vi "VNA and Opticool.vi"() -> ()   [LabVIEW 2024]
uses:
  <vilib>/Analysis/baseanly.llb/Mean (DBL).vi
  <vilib>/Utility/file.llb/Write Delimited Spreadsheet (DBL).vi
  <vilib>/Analysis/NI_AALBase.lvlib
  D:/LabData/Fan Fei/VNA/Agilent ENA Series/Agilent ENA Series.lvlib
panel:
  in  "file path":path=path "C:/Users/Public/OneDrive/Desktop/test/textR.txt"
  out "variance":dbl format="%0.2f"
  out "standard deviation":dbl format="%0.2f"
  out "mean":dbl=9.900000302096328e+37 format="%0.2f"
  in  "Num Meas":u32=10
  in  "Compliance  Level (0.1)":dbl=0.001
  in  "Source Mode  (0: Voltage)":u16(ring) items=["Voltage", "Current"]
  in  "Output Level (0)":dbl=3.0
  in  "VISA resource name 2":refnum<visa-resource-name>="GPIB0::18::INSTR"
  in  "stop":bool
  in  "file path (dialog if empty) Scan 2":path=path "C:/Users/B1172_SHG/Documents/NOEMS/test.txt"
  in  "Second Scan":bool
  in  "Port ( 1)  2":i32=1
  in  "Measurement Parameters   2":u16(ring)=1 items=["S11", "S21", "S31", "S41", "S12", "S22", "S32", "S42", "S13", "S23", "S33", "S43", "S14", "S24", "S34", "S44", "A", "B", "C", "D", "R1", "R2", "R3", "R4"]
  in  "Power Level (dBm)  2":dbl=-5.0 format="%^.2g"
  in  "VNA Points  2":i32=1000
  in  "Start (Mhz)  2":dbl=1.0 format="%^.2e"
  in  "Stop (MHz)  2":dbl=10.0 format="%^.2e"
  in  "Trigger Source   2":u16(ring) items=["Internal", "External", "Manual", "BUS"]
  in  "Point Trigger (F: Disable) 3":bool
  in  "Continuous Sweep (T: Enable)  2":bool=TRUE
  in  "Averaging State (F: Off) 3":bool
  in  "Average Factor (16) 3":i32=16
  in  "IF Bandwidth (100000.0)  2":dbl=1000.0 format="%^.1e"
  in  "Smoothing State (F: Off) 3":bool
  in  "Wait time (ms)  2":dbl=4000.0
  out "XY Graph 3":cluster{dbl[], "Primary / Real":dbl[]}(graph)
  in  "Continue":bool
  in  "Field Set when finsihed":dbl
  in  "Port ( 1)":i32=1
  in  "Measurement Parameters":u16(ring)=1 items=["S11", "S21", "S31", "S41", "S12", "S22", "S32", "S42", "S13", "S23", "S33", "S43", "S14", "S24", "S34", "S44", "A", "B", "C", "D", "R1", "R2", "R3", "R4"]
  in  "Power Level (dBm)":dbl=-5.0 format="%^.2g"
  in  "VNA Points":i32=1000
  in  "Start (Mhz)":dbl=1.0 format="%^.2e"
  in  "Stop (MHz)":dbl=10.0 format="%^.2e"
  in  "Trigger Source":u16(ring) items=["Internal", "External", "Manual", "BUS"]
  in  "Point Trigger (F: Disable) 2":bool
  in  "Continuous Sweep (T: Enable)":bool=TRUE
  in  "Averaging State (F: Off) 2":bool
  in  "Average Factor (16) 2":i32=16
  in  "IF Bandwidth (100000.0)":dbl=1000.0 format="%^.1e"
  in  "Smoothing State (F: Off) 2":bool
  in  "Wait time (ms)":dbl=4000.0
  out "XY Graph 2":cluster{dbl[], "Primary / Real":dbl[]}(graph)
  in  "T scan waiting time (min)":dbl
  in  "Scan T":bool=TRUE
  in  "T Step Size":dbl=10.0
  in  "Start B":dbl
  in  "B Step Size":dbl
  in  "B Number of Step":i32=1
  in  "Start T":dbl=300.0
  in  "T Number of Step":i32=20
  in  "Temperature Set when finish":dbl=300.0
  in  "file path (dialog if empty)":path=path "C:/Users/Public/OneDrive/Desktop/test/text.txt"
  in  "VISA resource name":refnum<visa-resource-name>="GPIB0::27::INSTR"
  in  "Remote":bool=TRUE
  in  "IP Address":string="169.254.170.239"
  out "Measuring":bool=TRUE
  out "Temperature":dbl=300.0
  in  "WaitForTemperature":bool=TRUE
  in  "WaitForField":bool=TRUE
  in  "Delay":dbl=5.0
  out "Field":dbl
  out "Field\nStatus":i32(ring)=4 items=["MagnetUnknown"=0, "StablePersistent"=1, "WarmingSwitch"=2, "CoolingSwitch"=3, "StableDriven"=4, "Iterating"=5, "Charging"=6, "Discharging"=7, "CurrentError"=8, "MagnetFailure"=15]
  out "Temperature\nStatus":i32(ring)=1 items=["TemperatureUnknown"=0, "Stable"=1, "Tracking"=2, "Near"=5, "Chasing"=6, "Filling"=7, "Standby"=10, "Disabled"=13, "ImpedanceNotFunction"=14, "TempFailure"=15]
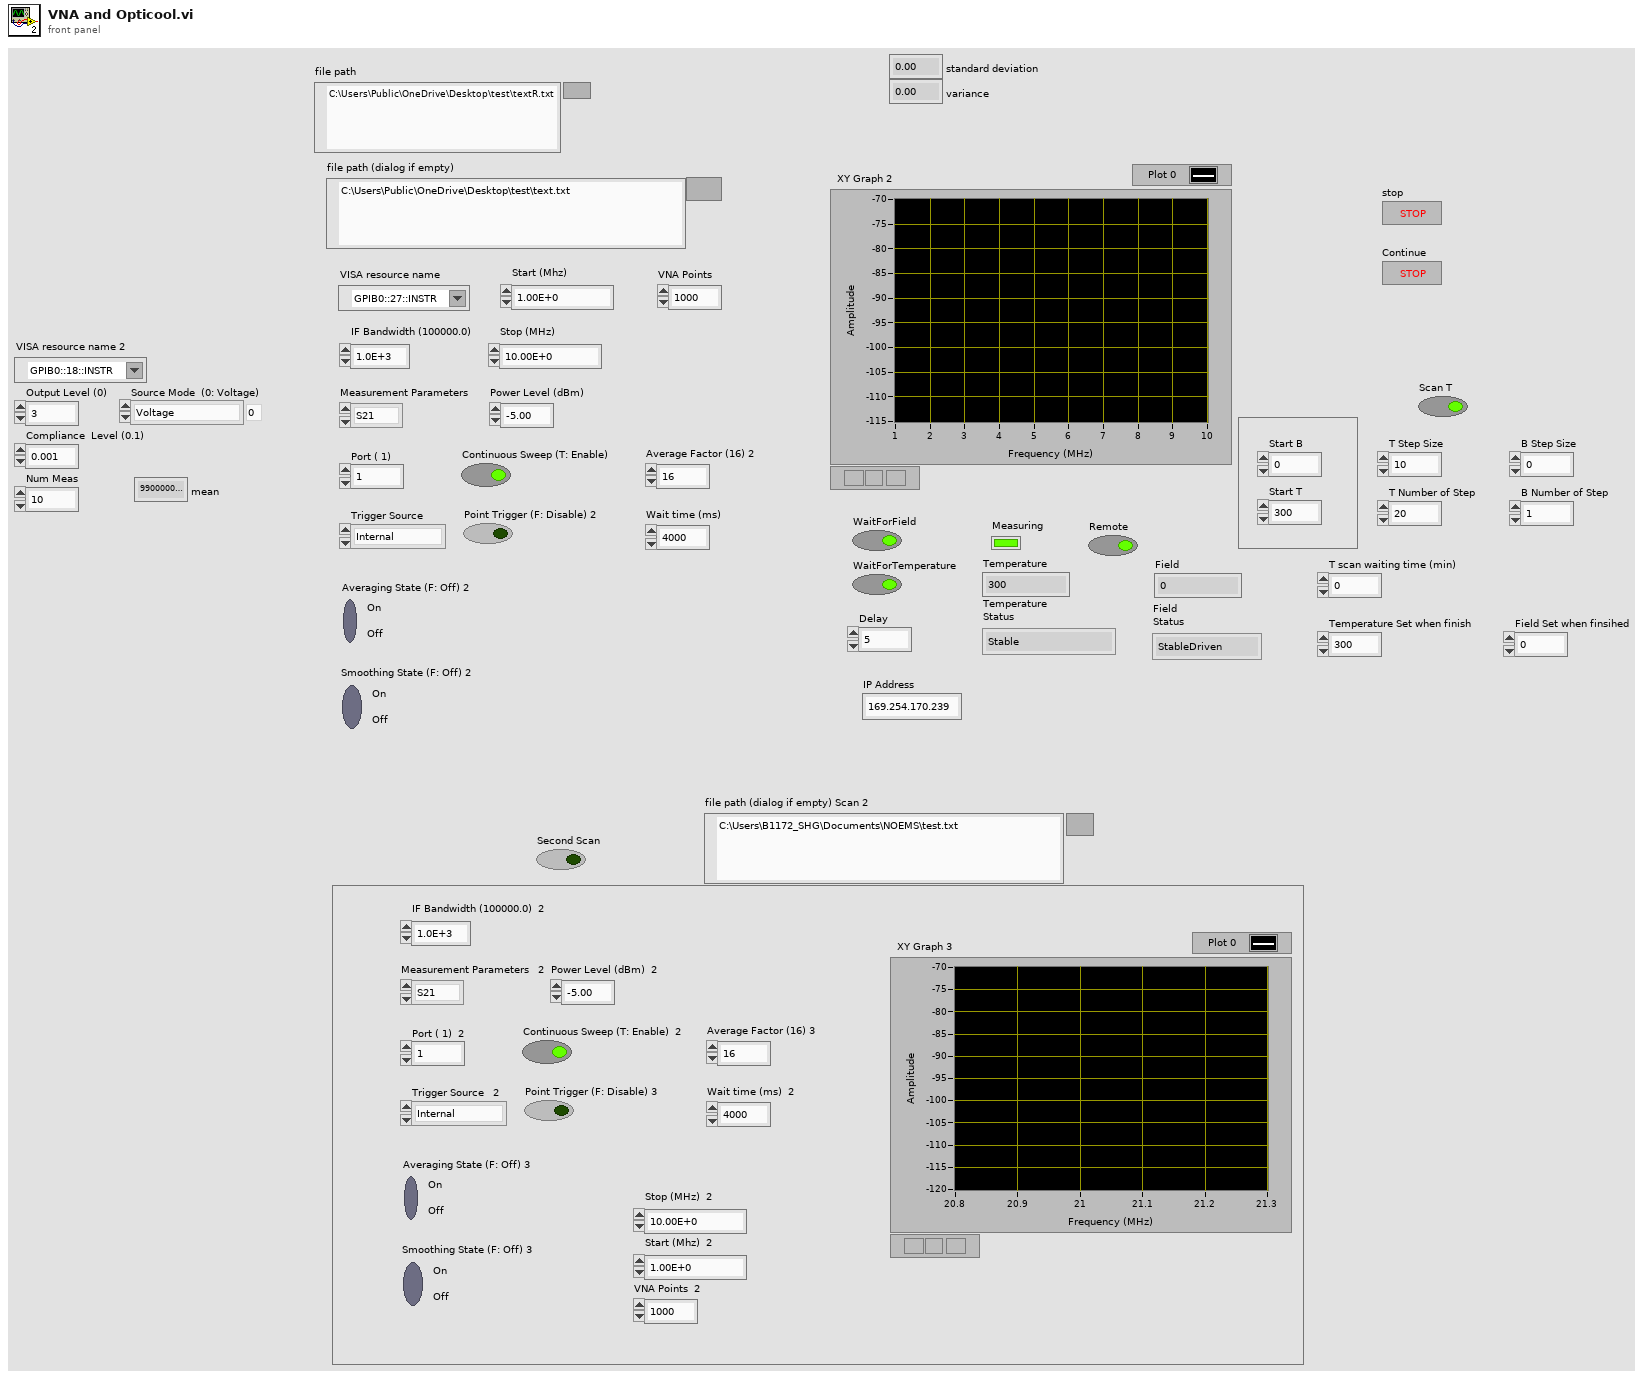
[diagram p1: front panel]
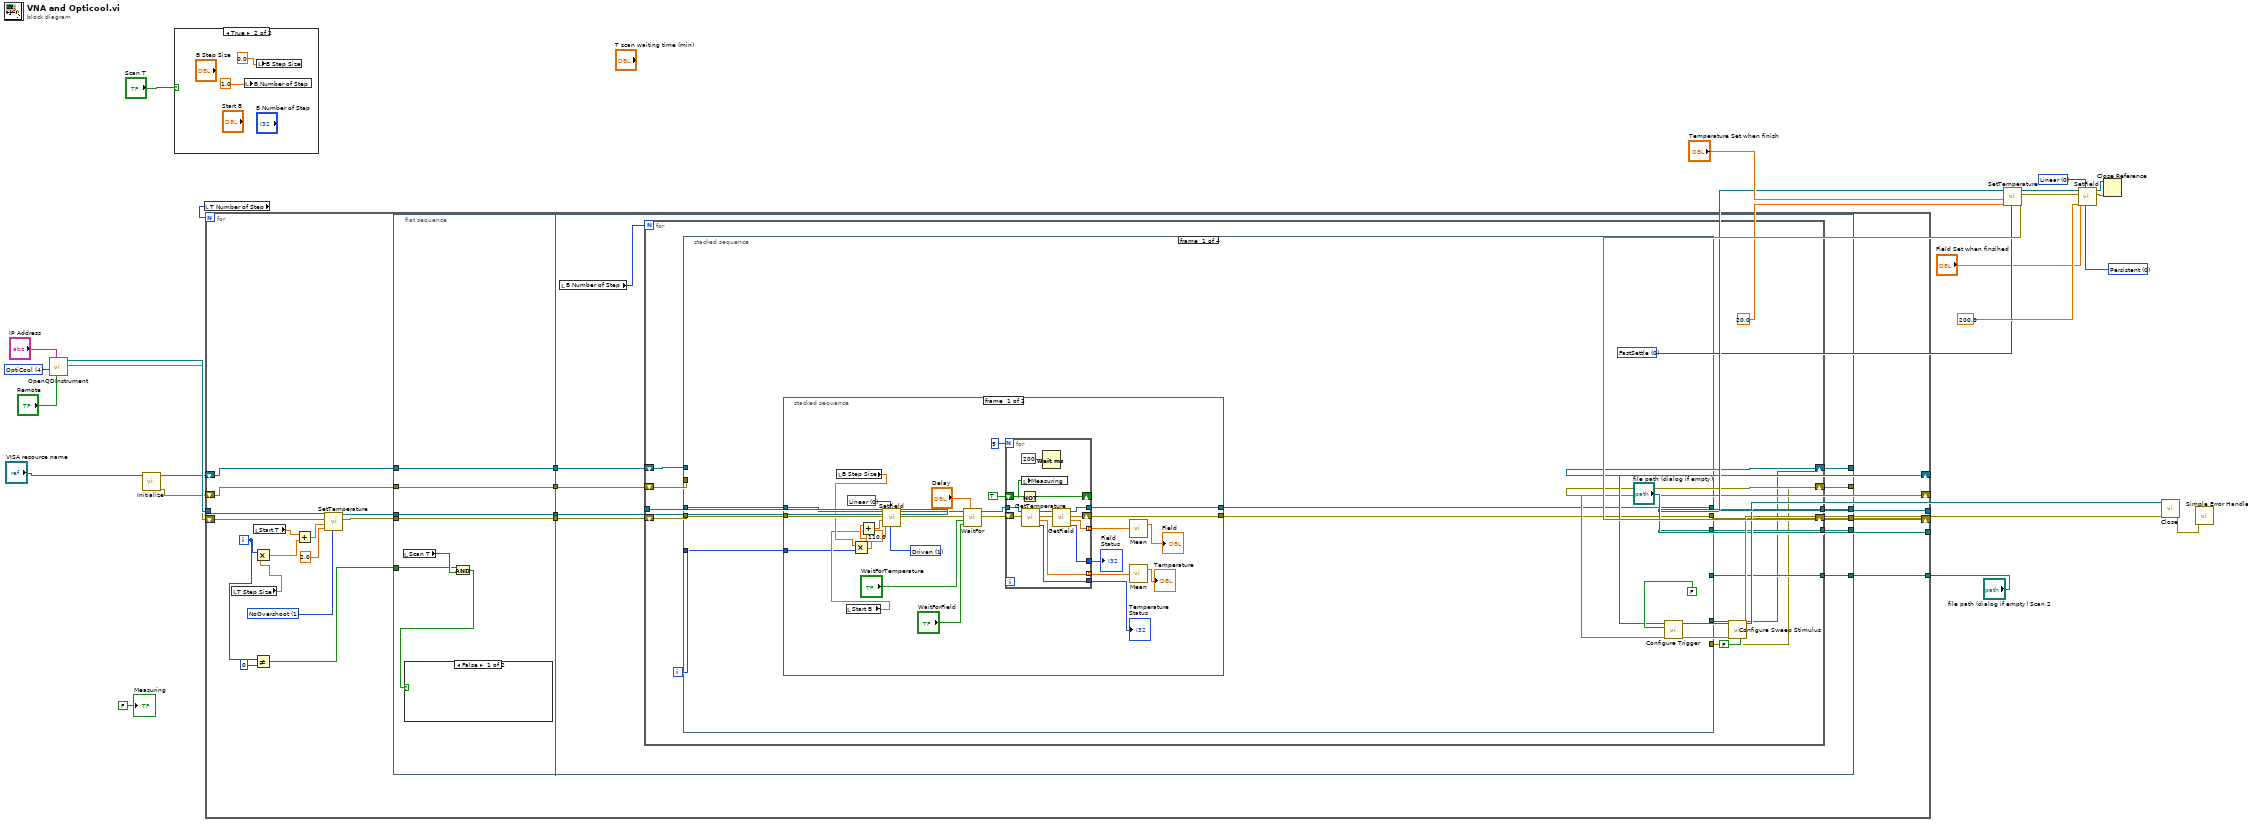
[diagram p0: block diagram]
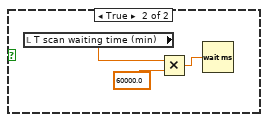
[diagram p2: hidden frame]
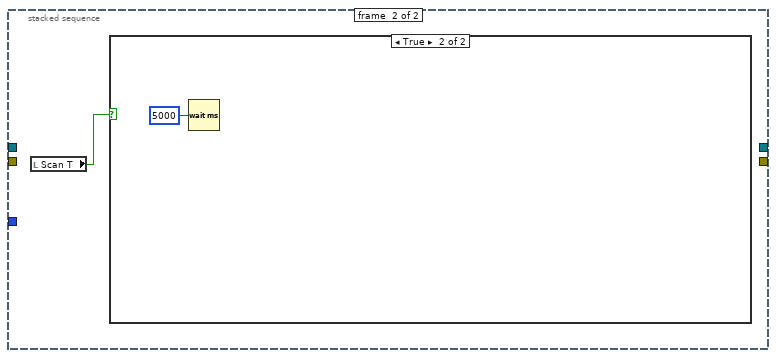
[diagram p3: hidden frame]
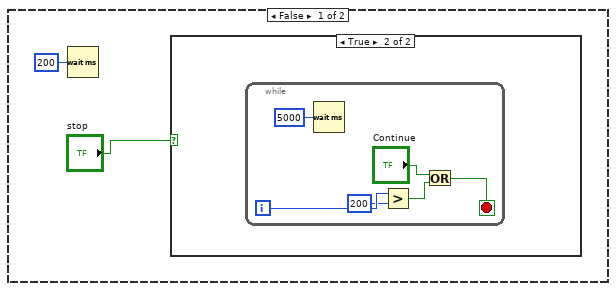
[diagram p4: hidden frame]
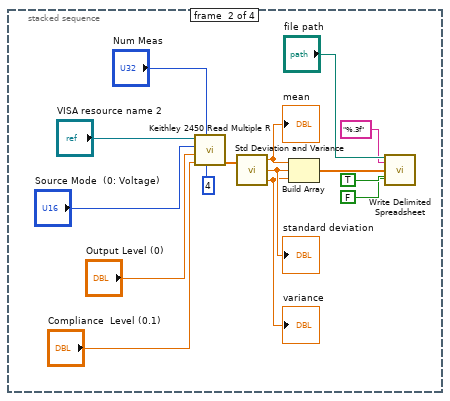
[diagram p6: hidden frame]
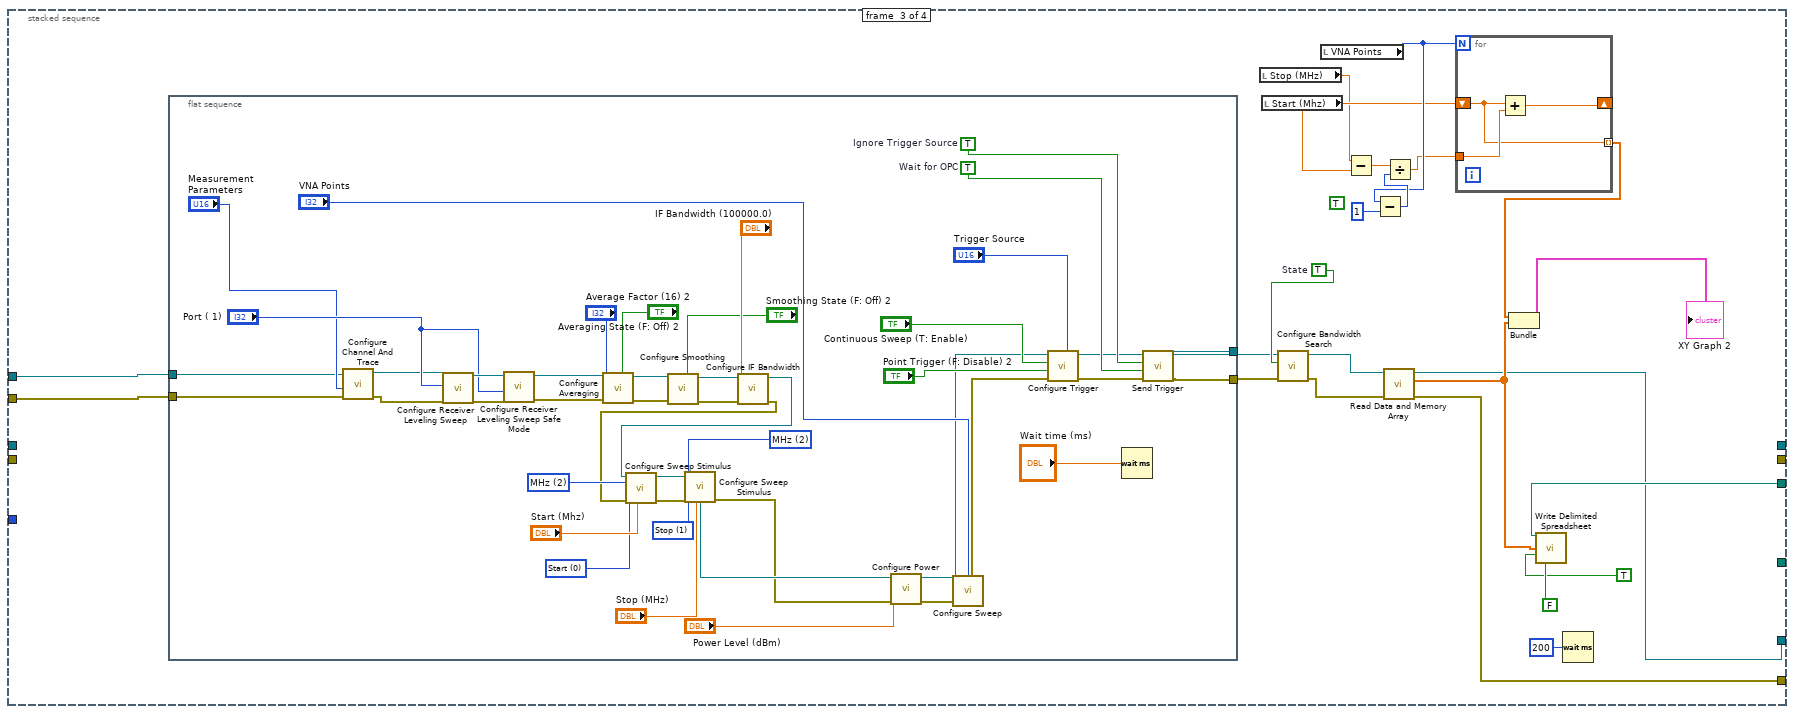
[diagram p7: hidden frame]
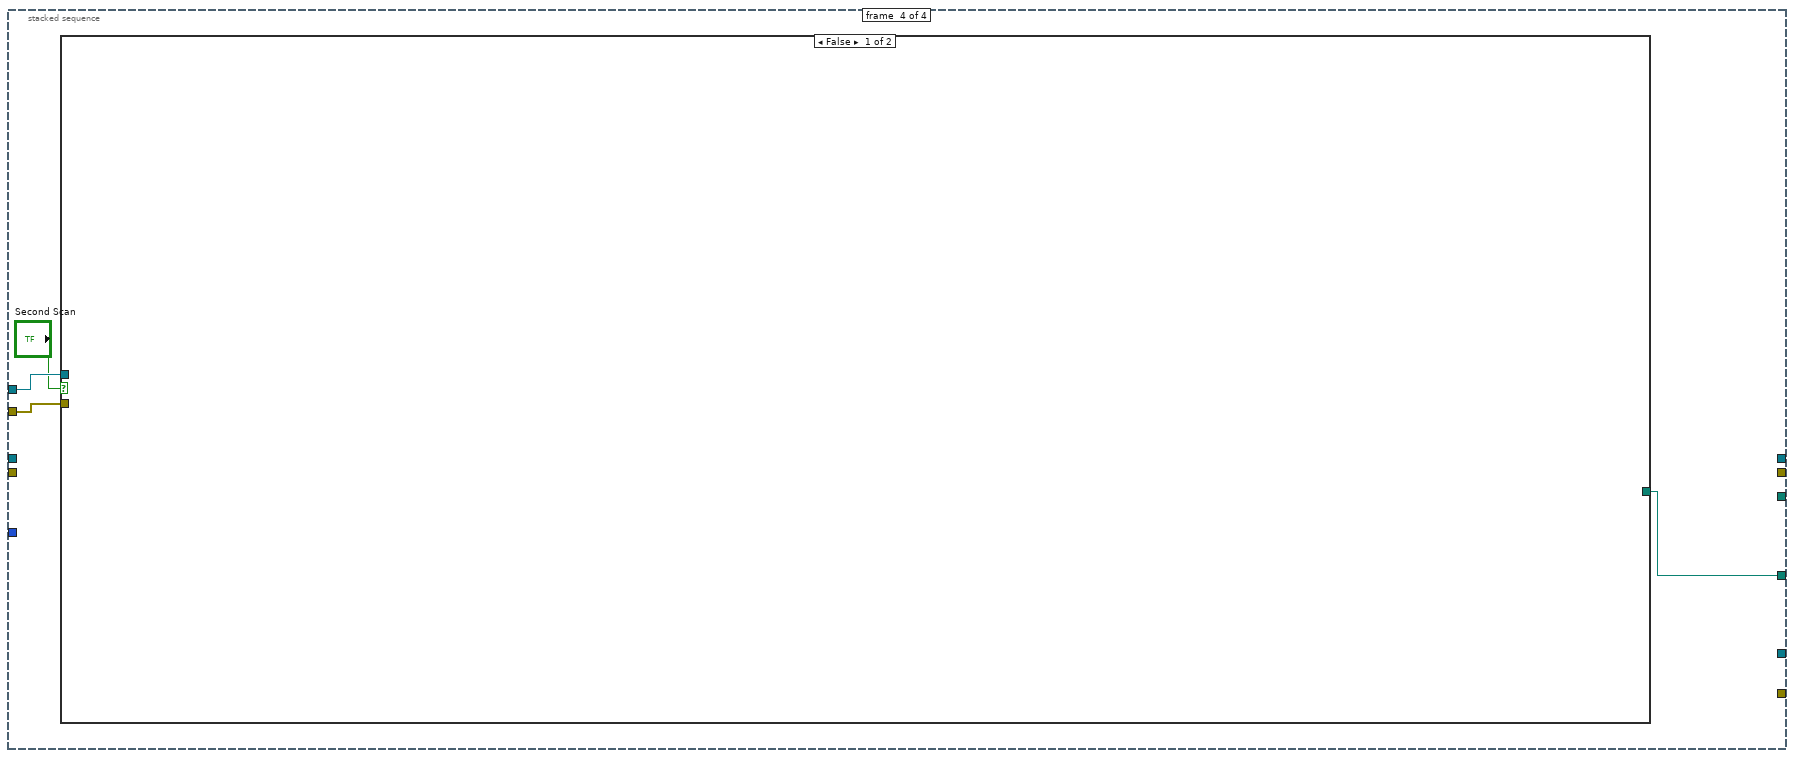
[diagram p8: hidden frame]
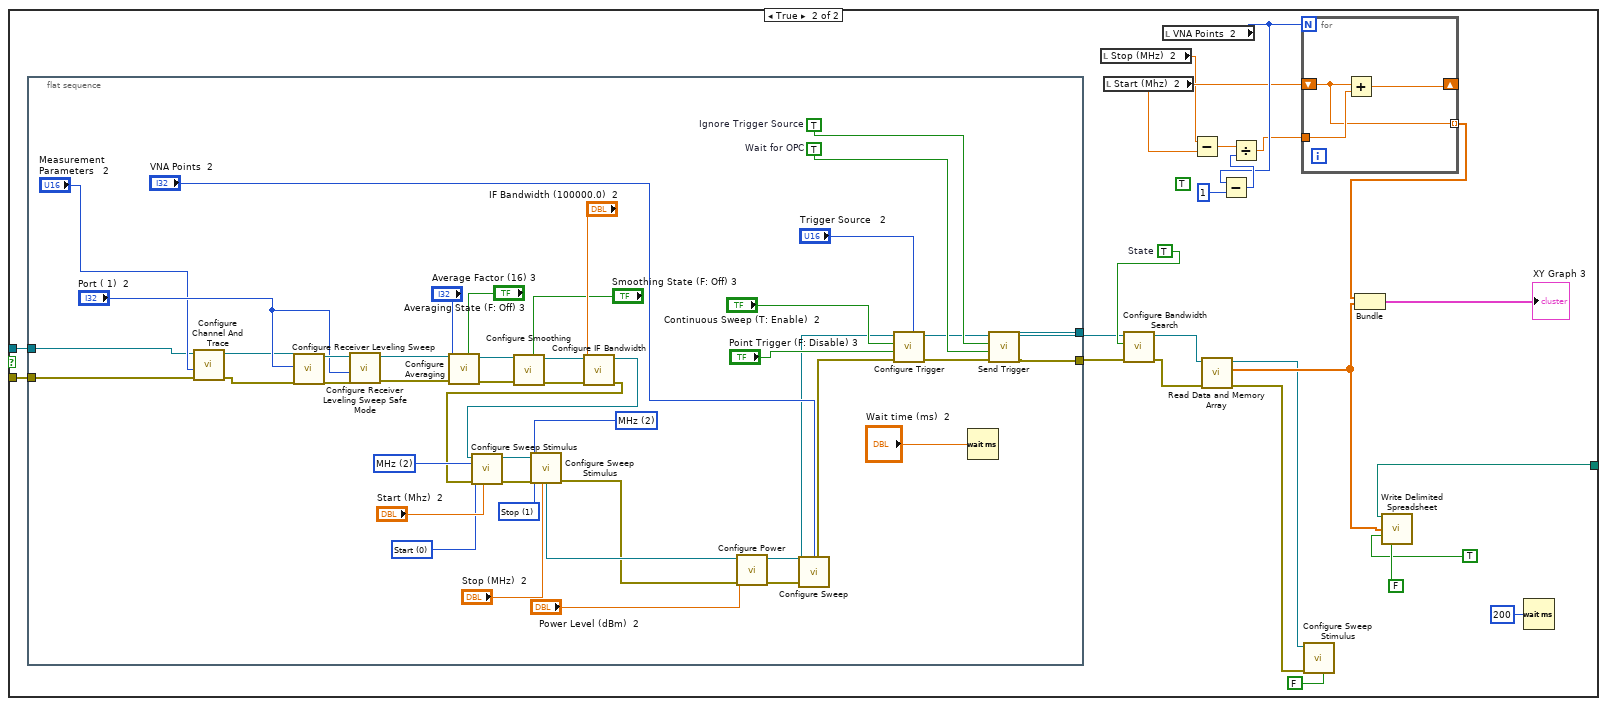
[diagram p9: hidden frame]
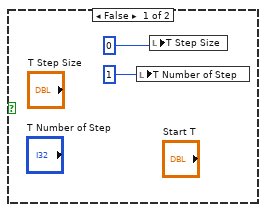
[diagram p10: hidden frame]
diagram:
  w18 = 0 items=["FastSettle", "NoOvershoot"] ("Approach")
  w21 = 4 items=["PPMS", "VersaLab", "DynaCool", "SVSM", "OptiCool"] ("InstrumentType")
  w33 = 0 items=["Persistent", "Driven"] ("Mode")
  w32 = 0 items=["Linear", "NoOvershoot", "Oscillate"] ("Approach")
  n1 = call "OpenQDInstrument.vi"("Remote"="Remote", "IP Address"="IP Address", "InstrumentType"=w21) -> ("error out"=w19:errorcluster, "Instrument Ref"=w20:refnum<k24>)  [unwired: 5 in]
  n2 = call "Initialize.vi"("VISA resource name"="VISA resource name") -> ("error out"=w3:errorcluster, "VISA resource name out"=w5:refnum<visa-resource-name>)  [unwired: 9 in]
  n3 = case shown="True" "Scan T" {
    frame False {
      n4 = local write "T Number of Step"(1) -> ()
      n5 = local write "T Step Size"(0) -> ()
    }
    frame True {
      n6 = local write "B Number of Step"(1.0 ("B Step Size")) -> ()
      n7 = local write "B Step Size"(0.0 ("B Step Size")) -> ()
    }
  }
  n8 = local read "T Number of Step"() -> (w8:i32)
  n9 = for {
    N: w8 -> [_]
    shift-right: [w58] -> w27
    shift-left: w19 -> [w62]
    tunnel: w20 -> [w61]
    tunnel: [w56] -> w24
    tunnel: "file path (dialog if empty)" -> [w52]
    shift-right: [w51] -> w7
    shift-left: w5 -> [w49]
    shift-right: [w50] -> w4
    shift-left: w3 -> [w48]
    tunnel: "file path (dialog if empty) Scan 2" -> [w43]
    i -> [w42]
    w57 = 1 items=["FastSettle", "NoOvershoot"] ("Approach")
    n10 = local read "T Step Size"() -> (w53:dbl)
    n11 = local read "Start T"() -> (w54:dbl)
    n12 = Multiply(x=w42, y=w53) -> (x*y=w55:dbl)
    n13 = Not Equal?(x=w42, y=0) -> (x != y?=w40:bool)
    n14 = Add(x=w54, y=w55) -> (x+y=w64:dbl)
    n15 = call "SetTemperature.vi"("Approach"=w57, "Rate"=2.0, "Temperature"=w64, "error in (no error)"=w62, "Instrument Ref In"=w61) -> ("error out"=w59:errorcluster, "Instrument Ref Out"=w60:refnum<k24>)  [unwired: 2 in, 1 out]
    n16 = flat-sequence {
      tunnel: w48 -> [w68]
      tunnel: w49 -> [w69]
      tunnel: w59 -> [w70]
      tunnel: w60 -> [w71]
      tunnel: [w71] -> w47
      tunnel: [w70] -> w46
      tunnel: [w69] -> w45
      tunnel: [w68] -> w44
      tunnel: w40 -> [w66]
      tunnel: [w83] -> w58
      tunnel: [w82] -> w56
      tunnel: w52 -> [w80]
      tunnel: [w79] -> w51
      tunnel: [w78] -> w50
      tunnel: w47 -> [w85]
      tunnel: w46 -> [w84]
      tunnel: w45 -> [w77]
      tunnel: w44 -> [w76]
      tunnel: w43 -> [w75]
      frame #0 {
        n17 = local read "Scan T"() -> (w67:bool)
        n18 = And(x=w66, y=w67) -> (x .and. y?=w65:bool)
        n19 = case shown="False" w65 {
          frame False {
          }
          frame True {
            n20 = local read "T scan waiting time (min)"() -> (w73:dbl)
            n21 = Multiply(x=w73, y=60000.0) -> (x*y=w72:dbl)
            n22 = Wait (ms)(milliseconds to wait=w72) -> ()  [unwired: 1 out]
          }
        }
      }
      frame #1 {
        n23 = local read "B Number of Step"() -> (w81:i32)
        n24 = for {
          N: w81 -> [_]
          tunnel: w85 -> [w96]
          shift-right: [w93] -> w83
          shift-left: w84 -> [w95]
          tunnel: [w94] -> w82
          tunnel: w80 -> [w92]
          shift-right: [w87] -> w79
          shift-left: w77 -> [w91]
          shift-right: [w86] -> w78
          shift-left: w76 -> [w90]
          tunnel: w75 -> [w88]
          i -> [w89]
          n25 = stacked-sequence {
            tunnel: w96 -> [w101 _ _ _]
            tunnel: w95 -> [w100 _ _ _]
            tunnel: [w99 _ _ _] -> w94
            tunnel: [w98 _ _ _] -> w93
            tunnel: w92 -> [_ _ w171 _]
            tunnel: [_ _ w170 _] -> w87
            tunnel: w91 -> [_ _ w169 w242]
            tunnel: w90 -> [_ _ w168 w241]
            tunnel: w89 -> [w97 _ _ _]
            tunnel: w88 -> [_ _ _ w239]
            tunnel: [_ _ w167 _] -> w86
            frame #0 {
              n26 = stacked-sequence {
                tunnel: w101 -> [w123 _]
                tunnel: w100 -> [w122 _]
                tunnel: [w115 _] -> w99
                tunnel: [w112 _] -> w98
                tunnel: w97 -> [w102 _]
                frame #0 {
                  w127 = 0 items=["Linear", "NoOvershoot", "Oscillate"] ("Approach")
                  w128 = 1 items=["Persistent", "Driven"] ("Mode")
                  n27 = local read "B Step Size"() -> (w107:dbl)
                  n28 = local read "Start B"() -> (w104:dbl)
                  n29 = Multiply(x=w107, y=w102) -> (x*y=w106:dbl)
                  n30 = Add(x=w106, y=w104) -> (x+y=w105:dbl)
                  n31 = call "SetField.vi"("Mode"=w128, "Approach"=w127, "Rate"=110.0, "Field"=w105, "error in (no error)"=w122, "Instrument Ref In"=w123) -> ("error out"=w121:errorcluster, "Instrument Ref Out"=w117:refnum<k24>)  [unwired: 1 in, 1 out]
                  n32 = call "WaitFor.vi"("Delay"="Delay", "Wait For Field"="WaitForField", "Wait For Temperature"="WaitForTemperature", "error in (no error)"=w121, "Instrument Ref In"=w117) -> ("error out"=w126:errorcluster, "Instrument Ref Out"=w116:refnum<k24>)  [unwired: 5 in]
                  n33 = for {
                    N: 5 -> [_]
                    shift-right: [w141] -> _
                    shift-left: TRUE -> [w139]
                    shift-right: [w136] -> w112
                    shift-left: w126 -> [w138]
                    tunnel: w116 -> [w135]
                    tunnel: [w133] -> w115
                    tunnel: [w130] -> w114
                    tunnel: [w129] -> w113
                    tunnel: [w131] -> w110 mode=indexing
                    tunnel: [w132] -> w111 mode=indexing
                    n34 = Not(x=w139) -> (.not. x?=w141:bool)
                    n35 = call "GetTemperature.vi"("error in (no error)"=w138, "Instrument Ref In"=w135) -> ("Temperature\nStatus"=w129:i32, "Temperature"=w132:dbl, "error out"=w137:errorcluster, "Instrument Ref Out"=w134:refnum<k24>)  [unwired: 3 in, 1 out]
                    n36 = local write "Measuring"(w139) -> ()
                    n37 = Wait (ms)(milliseconds to wait=u32 200) -> ()  [unwired: 1 out]
                    n38 = call "GetField.vi"("error in (no error)"=w137, "Instrument Ref In"=w134) -> ("Field\nStatus"=w130:i32, "Field"=w131:dbl, "error out"=w136:errorcluster, "Instrument Ref Out"=w133:refnum<k24>)  [unwired: 3 in, 1 out]
                  }
                  "Field\nStatus" <- w114
                  "Temperature\nStatus" <- w113
                  n39 = call-poly <vilib>:"Mean.vi"("X"=w110) -> ("mean"=→"Field":dbl)  [unwired: 1 out]
                  n40 = call-poly <vilib>:"Mean.vi"("X"=w111) -> ("mean"=→"Temperature":dbl)  [unwired: 1 out]
                }
                frame #1 {
                  n41 = local read "Scan T"() -> (w142:bool)
                  n42 = case shown="True" w142 {
                    frame False {
                      n43 = Wait (ms)(milliseconds to wait=u32 200) -> ()  [unwired: 1 out]
                      n44 = case shown="True" "stop" {
                        frame False {
                        }
                        frame True {
                          n45 = while {
                            i -> [w146]
                            stop <- w148 stop-if-true
                            n46 = Wait (ms)(milliseconds to wait=u32 5000) -> ()  [unwired: 1 out]
                            n47 = Greater?(x=w146, y=200) -> (0:w147:bool)
                            n48 = Or(x="Continue", y=w147) -> (x .or. y?=w148:bool)
                          }
                        }
                      }
                    }
                    frame True {
                      n49 = Wait (ms)(milliseconds to wait=u32 5000) -> ()  [unwired: 1 out]
                    }
                  }
                }
              }
            }
            frame #1 {
              n50 = call "Keithley 2450 Read Multiple R.vi"("num exclude"=u32 4, "Num Meas"="Num Meas", "Compliance  Level (0.1)"="Compliance  Level (0.1)", "Output Level (0)"="Output Level (0)", "Source Mode  (0: Voltage)"="Source Mode  (0: Voltage)", "VISA resource name"="VISA resource name 2") -> ("Resistance"=w154:sgl[])  [unwired: 5 in]
              n51 = call <vilib>:"Std Deviation and Variance.vi"("X"=w154) -> ("mean"=w165:dbl, "standard deviation"=w164:dbl, "variance"=w163:dbl)  [unwired: 1 in]
              "mean" <- w165
              "standard deviation" <- w164
              "variance" <- w163
              n52 = Build Array(w165, w164, w163) -> (w162:dbl[])
              n53 = call-poly <vilib>:"Write Delimited Spreadsheet.vi"("file path (dialog if empty)"="file path", "format (%.3f)"="%.3f", "1D data"=w162, "append to file? (new file:F)"=TRUE, "transpose? (no:F)"=FALSE) -> ()  [unwired: 9 in, 2 out]
            }
            frame #2 {
              w177 = TRUE  # State
              (unwired) TRUE ("Continuous Sweep (T: Enable)")
              n54 = flat-sequence {
                tunnel: [w193] -> w174
                tunnel: [w192] -> w173
                tunnel: w169 -> [w191]
                tunnel: w168 -> [w190]
                frame #0 {
                  w219 = u16 2 items=["Hz", "kHz", "MHz", "GHz", "dBm", "s", "V"] ("Unit (0: Hz)")
                  w220 = u16 2 items=["Hz", "kHz", "MHz", "GHz", "dBm", "s", "V"] ("Unit (0: Hz)")
                  w221 = u16 1 items=["Start", "Stop", "Center", "Span"] ("Stimulus (0: Start)")
                  w222 = u16 0 items=["Start", "Stop", "Center", "Span"] ("Stimulus (0: Start)")
                  w234 = TRUE  # Wait for OPC
                  w235 = TRUE  # Ignore Trigger Source
                  n55 = call "Configure Channel And Trace.vi"("error in (no error)"=w190, "Measurement Parameters (0: S11)"="Measurement Parameters", "VISA resource name"=w191) -> ("error out"=w205:errorcluster, "VISA resource name out"=w208:refnum<visa-resource-name>)  [unwired: 7 in]
                  n56 = call "Configure Receiver Leveling Sweep.vi"("VISA resource name"=w208, "Port ( 1)"="Port ( 1)", "error in (no error)"=w205) -> ("VISA resource name out"=w232:refnum<visa-resource-name>, "error out"=w204:errorcluster)  [unwired: 15 in]
                  n57 = call "Configure Receiver Leveling Sweep Safe Mode.vi"("error in (no error)"=w204, "Port ( 1)"="Port ( 1)", "VISA resource name"=w232) -> ("error out"=w203:errorcluster, "VISA resource name out"=w207:refnum<visa-resource-name>)  [unwired: 7 in]
                  n58 = call "Configure Averaging.vi"("Averaging State (F: Off)"="Averaging State (F: Off) 2", "error in (no error)"=w203, "Factor (16)"="Average Factor (16) 2", "VISA resource name"=w207) -> ("error out"=w202:errorcluster, "VISA resource name out"=w215:refnum<visa-resource-name>)  [unwired: 6 in]
                  n59 = call "Configure Smoothing.vi"("Smoothing State (F: Off)"="Smoothing State (F: Off) 2", "error in (no error)"=w202, "VISA resource name"=w215) -> ("error out"=w201:errorcluster, "VISA resource name out"=w214:refnum<visa-resource-name>)  [unwired: 7 in]
                  n60 = call "Configure IF Bandwidth.vi"("error in (no error)"=w201, "IF Bandwidth (100000.0)"="IF Bandwidth (100000.0)", "VISA resource name"=w214) -> ("error out"=w200:errorcluster, "VISA resource name out"=w213:refnum<visa-resource-name>)  [unwired: 7 in]
                  n61 = call "Configure Sweep Stimulus.vi"("Parameter (0.0)"="Start (Mhz)", "error in (no error)"=w200, "Stimulus (0: Start)"=w222, "Unit (0: Hz)"=w220, "VISA resource name"=w213) -> ("error out"=w199:errorcluster, "VISA resource name out"=w226:refnum<visa-resource-name>)  [unwired: 5 in]
                  n62 = call "Configure Sweep Stimulus.vi"("Parameter (0.0)"="Stop (MHz)", "error in (no error)"=w199, "Stimulus (0: Start)"=w221, "Unit (0: Hz)"=w219, "VISA resource name"=w226) -> ("error out"=w198:errorcluster, "VISA resource name out"=w225:refnum<visa-resource-name>)  [unwired: 5 in]
                  n63 = call "Configure Power.vi"("VISA resource name"=w225, "Power Level (0.0)"="Power Level (dBm)", "error in (no error)"=w198) -> ("VISA resource name out"=w228:refnum<visa-resource-name>, "error out"=w197:errorcluster)  [unwired: 11 in]
                  n64 = call "Configure Sweep.vi"("VISA resource name"=w228, "Number of Measurement Points (201)"="VNA Points", "error in (no error)"=w197) -> ("VISA resource name out"=w206:refnum<visa-resource-name>, "error out"=w196:errorcluster)  [unwired: 11 in]
                  n65 = call "Configure Trigger.vi"("Trigger Source (0: Internal)"="Trigger Source", "error in (no error)"=w196, "Point Trigger (F: Disable)"="Point Trigger (F: Disable) 2", "Continuous Sweep (T: Enable)"="Continuous Sweep (T: Enable)", "VISA resource name"=w206) -> ("error out"=w195:errorcluster, "VISA resource name out"=w233:refnum<visa-resource-name>)  [unwired: 5 in]
                  n66 = Wait (ms)(milliseconds to wait="Wait time (ms)") -> ()  [unwired: 1 out]
                  n67 = call "Send Trigger.vi"("error in (no error)"=w195, "Wait for OPC (F: Do not Wait)"=w234, "Ignore Trigger Source (F: Do not Ignore)"=w235, "VISA resource name"=w233) -> ("error out"=w192:errorcluster, "VISA resource name out"=w193:refnum<visa-resource-name>)  [unwired: 6 in]
                }
              }
              n68 = local read "Stop (MHz)"() -> (w182:dbl)
              n69 = local read "Start (Mhz)"() -> (w183:dbl)
              n70 = call "Configure Bandwidth Search.vi"("error in (no error)"=w173, "Result Display State (F: Disable)"=w177, "VISA resource name"=w174) -> ("error out"=w175:errorcluster, "VISA resource name out"=w176:refnum<visa-resource-name>)  [unwired: 7 in]
              n71 = local read "VNA Points"() -> (w186:i32)
              n72 = Subtract(x=w182, y=w183) -> (x-y=w184:dbl)
              n73 = Subtract(x=w186, y=1) -> (x-y=w187:i32)
              n74 = call "Read Data and Memory Array.vi"("error in (no error)"=w175, "VISA resource name"=w176) -> ("error out"=w167:errorcluster, "Primary / Real"=w172:dbl[], "VISA resource name out"=w170:refnum<visa-resource-name>)  [unwired: 6 in, 1 out]
              n75 = Divide(x=w184, y=w187) -> (x/y=w185:dbl)
              n76 = for {
                N: w186 -> [_]
                shift-right: [w238] -> _
                shift-left: w183 -> [w236]
                tunnel: w185 -> [w237]
                tunnel: [w236] -> w180 mode=indexing
                n77 = Add(x=w236, y=w237) -> (x+y=w238:dbl)
              }
              n78 = Bundle(w180, "Primary / Real"=w172) -> (→"XY Graph 2":cluster{dbl[], "Primary / Real":dbl[]})  [unwired: 1 in]
              n79 = call-poly <vilib>:"Write Delimited Spreadsheet.vi"("file path (dialog if empty)"=w171, "1D data"=w172, "append to file? (new file:F)"=TRUE, "transpose? (no:F)"=FALSE) -> ()  [unwired: 10 in, 2 out]
              n80 = Wait (ms)(milliseconds to wait=u32 200) -> ()  [unwired: 1 out]
            }
            frame #3 {
              n81 = case shown="False" "Second Scan" {
                tunnel: w242 -> [_ w248]
                tunnel: w241 -> [_ w247]
                tunnel: w239 -> [_ w246]
                frame False {
                }
                frame True {
                  w254 = TRUE  # State
                  (unwired) TRUE ("Continuous Sweep (T: Enable)")
                  n82 = flat-sequence {
                    tunnel: [w270] -> w251
                    tunnel: [w269] -> w250
                    tunnel: w248 -> [w268]
                    tunnel: w247 -> [w267]
                    frame #0 {
                      w296 = u16 2 items=["Hz", "kHz", "MHz", "GHz", "dBm", "s", "V"] ("Unit (0: Hz)")
                      w297 = u16 2 items=["Hz", "kHz", "MHz", "GHz", "dBm", "s", "V"] ("Unit (0: Hz)")
                      w298 = u16 1 items=["Start", "Stop", "Center", "Span"] ("Stimulus (0: Start)")
                      w299 = u16 0 items=["Start", "Stop", "Center", "Span"] ("Stimulus (0: Start)")
                      w311 = TRUE  # Wait for OPC
                      w312 = TRUE  # Ignore Trigger Source
                      n83 = call "Configure Channel And Trace.vi"("error in (no error)"=w267, "Measurement Parameters (0: S11)"="Measurement Parameters   2", "VISA resource name"=w268) -> ("error out"=w282:errorcluster, "VISA resource name out"=w285:refnum<visa-resource-name>)  [unwired: 7 in]
                      n84 = call "Configure Receiver Leveling Sweep.vi"("VISA resource name"=w285, "Port ( 1)"="Port ( 1)  2", "error in (no error)"=w282) -> ("VISA resource name out"=w309:refnum<visa-resource-name>, "error out"=w281:errorcluster)  [unwired: 15 in]
                      n85 = call "Configure Receiver Leveling Sweep Safe Mode.vi"("error in (no error)"=w281, "Port ( 1)"="Port ( 1)  2", "VISA resource name"=w309) -> ("error out"=w280:errorcluster, "VISA resource name out"=w284:refnum<visa-resource-name>)  [unwired: 7 in]
                      n86 = call "Configure Averaging.vi"("Averaging State (F: Off)"="Averaging State (F: Off) 3", "error in (no error)"=w280, "Factor (16)"="Average Factor (16) 3", "VISA resource name"=w284) -> ("error out"=w279:errorcluster, "VISA resource name out"=w292:refnum<visa-resource-name>)  [unwired: 6 in]
                      n87 = call "Configure Smoothing.vi"("Smoothing State (F: Off)"="Smoothing State (F: Off) 3", "error in (no error)"=w279, "VISA resource name"=w292) -> ("error out"=w278:errorcluster, "VISA resource name out"=w291:refnum<visa-resource-name>)  [unwired: 7 in]
                      n88 = call "Configure IF Bandwidth.vi"("error in (no error)"=w278, "IF Bandwidth (100000.0)"="IF Bandwidth (100000.0)  2", "VISA resource name"=w291) -> ("error out"=w277:errorcluster, "VISA resource name out"=w290:refnum<visa-resource-name>)  [unwired: 7 in]
                      n89 = call "Configure Sweep Stimulus.vi"("Parameter (0.0)"="Start (Mhz)  2", "error in (no error)"=w277, "Stimulus (0: Start)"=w299, "Unit (0: Hz)"=w297, "VISA resource name"=w290) -> ("error out"=w276:errorcluster, "VISA resource name out"=w303:refnum<visa-resource-name>)  [unwired: 5 in]
                      n90 = call "Configure Sweep Stimulus.vi"("Parameter (0.0)"="Stop (MHz)  2", "error in (no error)"=w276, "Stimulus (0: Start)"=w298, "Unit (0: Hz)"=w296, "VISA resource name"=w303) -> ("error out"=w275:errorcluster, "VISA resource name out"=w302:refnum<visa-resource-name>)  [unwired: 5 in]
                      n91 = call "Configure Power.vi"("VISA resource name"=w302, "Power Level (0.0)"="Power Level (dBm)  2", "error in (no error)"=w275) -> ("VISA resource name out"=w305:refnum<visa-resource-name>, "error out"=w274:errorcluster)  [unwired: 11 in]
                      n92 = call "Configure Sweep.vi"("VISA resource name"=w305, "Number of Measurement Points (201)"="VNA Points  2", "error in (no error)"=w274) -> ("VISA resource name out"=w283:refnum<visa-resource-name>, "error out"=w273:errorcluster)  [unwired: 11 in]
                      n93 = call "Configure Trigger.vi"("Trigger Source (0: Internal)"="Trigger Source   2", "error in (no error)"=w273, "Point Trigger (F: Disable)"="Point Trigger (F: Disable) 3", "Continuous Sweep (T: Enable)"="Continuous Sweep (T: Enable)  2", "VISA resource name"=w283) -> ("error out"=w272:errorcluster, "VISA resource name out"=w310:refnum<visa-resource-name>)  [unwired: 5 in]
                      n94 = Wait (ms)(milliseconds to wait="Wait time (ms)  2") -> ()  [unwired: 1 out]
                      n95 = call "Send Trigger.vi"("error in (no error)"=w272, "Wait for OPC (F: Do not Wait)"=w311, "Ignore Trigger Source (F: Do not Ignore)"=w312, "VISA resource name"=w310) -> ("error out"=w269:errorcluster, "VISA resource name out"=w270:refnum<visa-resource-name>)  [unwired: 6 in]
                    }
                  }
                  n96 = local read "Stop (MHz)  2"() -> (w259:dbl)
                  n97 = local read "Start (Mhz)  2"() -> (w260:dbl)
                  n98 = call "Configure Bandwidth Search.vi"("error in (no error)"=w250, "Result Display State (F: Disable)"=w254, "VISA resource name"=w251) -> ("error out"=w252:errorcluster, "VISA resource name out"=w253:refnum<visa-resource-name>)  [unwired: 7 in]
                  n99 = local read "VNA Points  2"() -> (w263:i32)
                  n100 = Subtract(x=w259, y=w260) -> (x-y=w261:dbl)
                  n101 = call "Read Data and Memory Array.vi"("error in (no error)"=w252, "VISA resource name"=w253) -> ("error out"=w245:errorcluster, "Primary / Real"=w249:dbl[], "VISA resource name out"=w244:refnum<visa-resource-name>)  [unwired: 6 in, 1 out]
                  n102 = Subtract(x=w263, y=1) -> (x-y=w264:i32)
                  n103 = Divide(x=w261, y=w264) -> (x/y=w262:dbl)
                  n104 = for {
                    N: w263 -> [_]
                    shift-right: [w315] -> _
                    shift-left: w260 -> [w313]
                    tunnel: w262 -> [w314]
                    tunnel: [w313] -> w257 mode=indexing
                    n105 = Add(x=w313, y=w314) -> (x+y=w315:dbl)
                  }
                  n106 = call "Configure Sweep Stimulus.vi"("Signal Output (T: On)"=FALSE, "error in (no error)"=w245, "VISA resource name"=w244) -> ()  [unwired: 7 in, 2 out]
                  n107 = Bundle(w257, "Primary / Real"=w249) -> (→"XY Graph 3":cluster{dbl[], "Primary / Real":dbl[]})  [unwired: 1 in]
                  n108 = call-poly <vilib>:"Write Delimited Spreadsheet.vi"("file path (dialog if empty)"=w246, "1D data"=w249, "append to file? (new file:F)"=TRUE, "transpose? (no:F)"=FALSE) -> ()  [unwired: 10 in, 2 out]
                  n109 = Wait (ms)(milliseconds to wait=u32 200) -> ()  [unwired: 1 out]
                }
              }
            }
          }
        }
      }
    }
  }
  n110 = call "Configure Trigger.vi"("error in (no error)"=w4, "Continuous Sweep (T: Enable)"=FALSE, "VISA resource name"=w7) -> ("error out"=w12:errorcluster, "VISA resource name out"=w13:refnum<visa-resource-name>)  [unwired: 7 in]
  n111 = call "Configure Sweep Stimulus.vi"("Signal Output (T: On)"=FALSE, "error in (no error)"=w12, "VISA resource name"=w13) -> ("error out"=w15:errorcluster, "VISA resource name out"=w16:refnum<visa-resource-name>)  [unwired: 7 in]
  n112 = call "SetTemperature.vi"("Approach"=w18, "Rate"=20.0, "Temperature"="Temperature Set when finish", "error in (no error)"=w27, "Instrument Ref In"=w24) -> ("error out"=w30:errorcluster, "Instrument Ref Out"=w29:refnum<k24>)  [unwired: 2 in, 1 out]
  n113 = call "SetField.vi"("Mode"=w33, "Approach"=w32, "Rate"=200.0, "Field"="Field Set when finsihed", "error in (no error)"=w30, "Instrument Ref In"=w29) -> ("error out"=w35:errorcluster, "Instrument Ref Out"=w34:refnum<k24>)  [unwired: 1 in, 1 out]
  n114 = Close Reference(reference=w34, error in (no error)=w35) -> ()  [unwired: 1 out]
  n115 = call "Close.vi"("error in (no error)"=w15, "VISA resource name"=w16) -> ("error out"=w17:errorcluster)  [unwired: 9 in]
  n116 = call <vilib>:"Simple Error Handler.vi"("error in (no error)"=w17) -> ()  [unwired: 4 in, 5 out]
  "Measuring" <- FALSE
